vi "NEW LOAD CELL PID.vi"(8 "error in (no error)":errorcluster, 10 "Checkbox":bool, 11 "main ref":T1) -> (0 "error out":errorcluster)   [LabVIEW 2025]
uses:
  controls/LAB-IQ UI Data.ctl
  HEAVE vi's/Heave Write enum.ctl
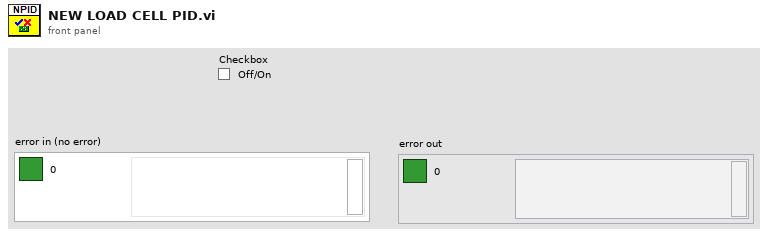
[diagram p1: front panel]
types:
  T1 = typedef "LAB-IQ UI Data.ctl" = cluster{"Main Home Screen":cluster{"GUI":refnum<vi>, "Platform Settings":refnum<vi>, "Configure":refnum<vi>, "Home":refnum<vi>, "EXIT":refnum<vi>, "service 2":refnum<vi>, "MainPage":refnum<vi>, "Analysis":refnum<vi>}, "Platform Settings":cluster{"mm/s  Surge":refnum<vi>, "Update Surge Speed":refnum<vi>, "Drive Error":refnum<vi>, "Disable Axis Jog Soft Limits":refnum<vi>, "mm/s  Sway":refnum<vi>, "Sway and Surge COM Status":refnum<vi>, "Heave COM Status":refnum<vi>, "Enable Platform":refnum<vi>, "Surge Forward Main":refnum<vi>, "Sway Right Main":refnum<vi>, "Sway Left Main":refnum<vi>, "Heave Down Main":refnum<vi>, "Heave Up main":refnum<vi>, "Update Sway Speed":refnum<vi>, "Update Heave Speed":refnum<vi>, "mm/s Heave":refnum<vi>, "mm/sec":refnum<vi>, "mm":refnum<vi>, "Surge Backward Main":refnum<vi>}, "Analysis Screen":cluster{"Analysis Home":refnum<vi>, "Surface Analysis":refnum<vi>, "Imaging":refnum<vi>, "Image Analysis":refnum<vi>, "Post Analysis":refnum<vi>}, "Config Screen":cluster{"Select Load Head":refnum<vi>, "Notes :":refnum<vi>, "FILE":refnum<vi>, "Sample ID :":refnum<vi>, "Operator ID :":refnum<vi>, "Operator Name :":refnum<vi>, "Auto":refnum<vi>}, "Motion Module":cluster{"zNL":refnum<vi>, "NL disp":refnum<vi>, "Rotary Tab":refnum<vi>, "Motion Direction:  3":refnum<vi>, "E.Velocity 2":refnum<vi>, "e.v/ssr 2":refnum<vi>, "Enter Fixed E.Velocity 2":refnum<vi>, "Enter Final SRR 2":refnum<vi>, "Enter initial SRR 2":refnum<vi>, "Enter Fixed SRR 2":refnum<vi>, "Enter the Final E.Velocity (m/s) 2":refnum<vi>, "Enter initial E.Velocity (m/s) 2":refnum<vi>, "Final Speed (RPM) 3":refnum<vi>, "Initial Speed (RPM) 2":refnum<vi>, "Enter the Final Velocity (m/s) 3":refnum<vi>, "Enter initial Velocity (m/s)  3":refnum<vi>, "Ramp Up 2":refnum<vi>, "TEST SELECTION":refnum<vi>, "SPEED SELECTION : ":refnum<vi>, "Angular Oscillation Set":refnum<vi>, "Traction":refnum<vi>, "Step Speed":refnum<vi>, "StepTable For Load-Speed":refnum<vi>, "StepTable For Speed":refnum<vi>, "Surge Forward MM":refnum<vi>, "Surge Backward MM":refnum<vi>, "M3 Image":refnum<vi>, "String 39":refnum<vi>, "Sway Left MM":refnum<vi>, "Sway Right MM":refnum<vi>, "Disable Axis Jog Soft Limits":refnum<vi>, "mm":refnum<vi>, "Heave Down MM":refnum<vi>, "Heave Up MM":refnum<vi>, "Wear Track Diameter (mm)":refnum<vi>, "Set WTD":refnum<vi>, "HomeScratch":refnum<vi>, "HomeRot":refnum<vi>, "PlaceModule":refnum<vi>, "Enter the Angle (Deg)":refnum<vi>, "Enter the Frequency (Hz)":refnum<vi>, "Motion Mode:":refnum<vi>, "LR Sway":refnum<vi>, "Rot Hor":refnum<vi>, "Scratch":refnum<vi>, "LR Cam":refnum<vi>, "MMBack":refnum<vi>, "MMNext":refnum<vi>, "Rot Ver":refnum<vi>, "Rotary Module Selection":refnum<vi>, "calculate rotary":refnum<vi>, "SPEED SELECTION : rotary":refnum<vi>, "Import 2":refnum<vi>, "Save 2":refnum<vi>, "File Path :  2":refnum<vi>, "String 45":refnum<vi>, "StepTable For Speed 3":refnum<vi>, "Enter the Speed(mm/sec)":refnum<vi>, "Enter the Speed(RPM)":refnum<vi>, "Enter Scratch Speed (mm/s):":refnum<vi>, "SwaySpeed Set":refnum<vi>, "Scartch Offset":refnum<vi>, "Motion type:":refnum<vi>, "HomeScratch 2":refnum<vi>, "Enter Scratch length (mm):":refnum<vi>, "Wear Track Diameter":refnum<vi>, "Rotary Speed Exced":refnum<vi>, "Scratch Mode":refnum<vi>, "No of Scratch":refnum<vi>}, "Environmental control":cluster{"Humidity  Status  3":refnum<vi>, "Low Temp  Status  2":refnum<vi>, "TK4 status 2":refnum<vi>, "Stage Temperature":refnum<vi>, "Sample Temperature":refnum<vi>, "Humidity (Amb)":refnum<vi>, "Clear List":refnum<vi>, "Add to list":refnum<vi>, "Wear":refnum<vi>, "Vibration":refnum<vi>, "Humidity (Chamber)":refnum<vi>, "Temperature (Chamber)":refnum<vi>, "ECR ":refnum<vi>, "Temperature (Amb)":refnum<vi>, "Microphone":refnum<vi>, "Acoustic Emission 3":refnum<vi>, "SNext":refnum<vi>, "APBack":refnum<vi>, "Enter the Temperature (°C):":refnum<vi>, "Enter the Stage \nTemperature (°C):":refnum<vi>, "Enter the Humidity (%Rh):":refnum<vi>, "Low Temp":refnum<vi>, "High Temp":refnum<vi>, "Humidity":refnum<vi>, "Sensors Picked":refnum<vi>}, "About Screen":cluster{"Password":refnum<vi>, "Home Service":refnum<vi>, "Advanced Setting":refnum<vi>, "About Tab":refnum<vi>, "ECR Port:":refnum<vi>, "Ramp Port:":refnum<vi>, "Installation/Replacement completed":refnum<vi>, "Loahead":refnum<vi>, "Heave and Surge COM Port:":refnum<vi>, "Sway COM Port:":refnum<vi>, "Temp Modbus:":refnum<vi>, "Humidity Port:":refnum<vi>, "Edit Gain Constants":refnum<vi>, "Save Gain Constants":refnum<vi>}, "Main Screen":cluster{"Main Screen Tab":refnum<vi>, "Angle and Frequency":refnum<vi>, "Stroke (mm)":refnum<vi>, "Angle (Deg)":refnum<vi>, "Main Speed Tab":refnum<vi>, "MTM MOTOR DISPLAY":refnum<vi>, "Disc Speed (m/sec)":refnum<vi>, "Ball Speed (m/sec)":refnum<vi>, "Disc Speed (RPM)":refnum<vi>, "Ball Speed (RPM)":refnum<vi>, "SPEED TAB":refnum<vi>, "Speed (m/sec)":refnum<vi>, "Set Speed (m/sec)":refnum<vi>, "Speed (RPM)":refnum<vi>, "Set Speed":refnum<vi>, "Time Tab":refnum<vi>, "Time ( HH:MM:SS ) 2":refnum<vi>, "Test Duration":refnum<vi>, "Test Duration 4":refnum<vi>, "TEST CYCLE":refnum<vi>, "TOTAL CYCLES":refnum<vi>, "Set Load (N)":refnum<vi>, "Temp Tabs":refnum<vi>, "Heater":refnum<vi>, "TK4 status":refnum<vi>, "ChamberTemp":refnum<vi>, "SetTmp":refnum<vi>, "Controller  Status":refnum<vi>, "ChamberTemp 2":refnum<vi>, "SetTmp 2":refnum<vi>, "Controller  Status 2":refnum<vi>, "ChamberTemp 3":refnum<vi>, "SetTmp 3":refnum<vi>, "Cooling":refnum<vi>, "Load Communication":refnum<vi>, "Ambient \nTemperature":refnum<vi>, "HumCOMStatus":refnum<vi>, "Ambient\n Humidity":refnum<vi>, "Freq (Hz)":refnum<vi>, "Load En":refnum<vi>, "NLt":refnum<vi>, "zNL 2":refnum<vi>, "Humidity On":refnum<vi>, "humidity disp":refnum<vi>, "Set Humidity":refnum<vi>, "NL disp 2":refnum<vi>, "Humidity On 2":refnum<vi>, "humidity disp 2":refnum<vi>, "Set Humidity 2":refnum<vi>, "NL disp 3":refnum<vi>, "AppLoadSeq scratch":refnum<vi>, "Stop Scratch":refnum<vi>, "ClrLog":refnum<vi>, "Trip Log":refnum<vi>, "STOP":refnum<vi>, "Start Test":refnum<vi>, "Test status":refnum<vi>, "AR Led":refnum<vi>, "Data":refnum<vi>, "Health":refnum<vi>, "Sway COM Status":refnum<vi>, "Heave COM Status":refnum<vi>, "Grp Tab":refnum<vi>, "Sub Graph":refnum<vi>, "SD (mm)":refnum<vi>, "Siliding distance Reset Graph":refnum<vi>, "SDGp":refnum<vi>, "Humidity Reset Graph":refnum<vi>, "HumrGp":refnum<vi>, "Acoustic Emission (mV)":refnum<vi>, "Aqucostic Reset Graph":refnum<vi>, "gACQUOS":refnum<vi>, "ECR RESET":refnum<vi>, "ECR":refnum<vi>, "Temperature Reset":refnum<vi>, "Acoustic Emission (mV) 2":refnum<vi>, "Aqucostic Reset Graph 2":refnum<vi>, "gACQUOS 2":refnum<vi>, "ECR RESET 2":refnum<vi>, "ECR 2":refnum<vi>, "Temperature Reset 2":refnum<vi>, "Temperature (deg c)":refnum<vi>, "Speed Reset Graph":refnum<vi>, "Speed Tab":refnum<vi>, "MTM DISC  SPEED":refnum<vi>, "MTM BALL SPEED":refnum<vi>, "speed mm/sec":refnum<vi>, "Hymidity":refnum<vi>, "Humidity Disable trip":refnum<vi>, "CoF Trip  2":refnum<vi>, "Depth Trip":refnum<vi>, "Weart Deapth":refnum<vi>, "Depth Reset Graph":refnum<vi>, "Weart":refnum<vi>, "Depthz":refnum<vi>, "Depth (µm)":refnum<vi>, "WearGp":refnum<vi>, "NL Trip 2":refnum<vi>, "Load pid":refnum<vi>, "Load Disable Trip":refnum<vi>, "Load Reset Graph":refnum<vi>, "NL Display 4":refnum<vi>, "Main Chart 3":refnum<vi>, "BACK":refnum<vi>, "Depth Trip 2":refnum<vi>, "COF TRIP ":refnum<vi>, "Friction Force (N)":refnum<vi>, "FF Reset Graph":refnum<vi>, "FF Disable Trip":refnum<vi>, "FF TRIP":refnum<vi>, "COF Disable Trip":refnum<vi>, "COF Reset Graph":refnum<vi>, "Start Test Temp":refnum<vi>, "zFF":refnum<vi>, "Friction Force (N) Graph":refnum<vi>, "Coefficient of Friction":refnum<vi>, "Scratch Start Test":refnum<vi>, "FF Tab":refnum<vi>, "Cyclic Friction Force (N)":refnum<vi>, "CZ FF":refnum<vi>, "Cyclic Friction Force (N) Graph":refnum<vi>, "Cyclic Coefficient of Friction":refnum<vi>, "Cyclic FF TRIP":refnum<vi>, "Cyclic FF Disable Trip":refnum<vi>, "cyclic COF Disable Trip":refnum<vi>, "cyclic COF TRIP":refnum<vi>, "cyclic COF Reset Graph":refnum<vi>, "Cyclic FF Reset Graph":refnum<vi>, "Test Trip":refnum<vi>, "Multi Scratch Pass":refnum<vi>}, "Loading":cluster{"Indentation":refnum<vi>, "Reference Sample":refnum<vi>, "Load Cell Communication Slide":refnum<vi>, "com 3":refnum<vi>, "com":refnum<vi>, "DecaForce COM Status":refnum<vi>, "Update":refnum<vi>, "Clear 3":refnum<vi>, "seq":refnum<vi>, "Stribeck table":refnum<vi>, "Stribeck Table  For loading":refnum<vi>, "Loading Mode":refnum<vi>, "Enter the Final Load (N)":refnum<vi>, "Enter the CoF Trip":refnum<vi>, "Enter the Friction Force Trip":refnum<vi>, "Enter the Normal load Trip":refnum<vi>, "Enter the Load  (N)":refnum<vi>, "KiloForce":refnum<vi>, "DecaForce ":refnum<vi>, "MicroForce":refnum<vi>, "LHBack":refnum<vi>, "LHNext":refnum<vi>, "Enter the Loading Rate (N/min)":refnum<vi>, "Message":refnum<vi>, "Warning 2":refnum<vi>, "SSP 0.75":refnum<vi>, "SSP 0.5":refnum<vi>, "SSP 0.3":refnum<vi>, "Warning":refnum<vi>, "gui GIF":refnum<vi>, "Communication is established":refnum<vi>, "AppLoad 4":refnum<vi>, "Multipoint":refnum<vi>, "Load Selection":refnum<vi>}, "PID":cluster{"Ramp MulFac":refnum<vi>, "pulses LoadDiffRamp(2..10)":refnum<vi>, "PulseControlRamp(diff<=3N)":refnum<vi>, "SetLoadDeadband(%) Load(0-10N)":refnum<vi>, "PID gains out delay (microForce)":refnum<vi>, "Ramp":refnum<vi>, "Gain 2":refnum<vi>, "pulses LoadDiff(2..10)":refnum<vi>, "pulses LoadDiff(11..50)":refnum<vi>, "PulseControl(diff<=3N)":refnum<vi>, "SetLoadDeadband(%)  2":refnum<vi>, "Dummy Run":refnum<vi>, "Vertical load (N)":refnum<vi>, "AutoTune":refnum<vi>, "Offset 3 ":refnum<vi>, "apply load":refnum<vi>, "Offset  3":refnum<vi>, "apply load 2":refnum<vi>, "Enter ByPass Load":refnum<vi>, "reinit 3":refnum<vi>, "output range delay":refnum<vi>, "PID gains out delay":refnum<vi>, "Bypass Load":refnum<vi>, "pulsesSent":refnum<vi>, "pulses ":refnum<vi>, "actpid":refnum<vi>, "gFF Rot":refnum<vi>, "pulses LoadDiff(21..1000)":refnum<vi>, "Delay":refnum<vi>, "deadband":refnum<vi>}, "Config Parameters":cluster{"Tab Control 3":refnum<vi>, "Tab Control 19":refnum<vi>, "SAMPLES":refnum<vi>, "Re-initilaize":refnum<vi>, "Filter ON/OFF":refnum<vi>, "TracHomeSurgeOffsetCounts 10MM":refnum<vi>, "TracHomeSwayOffsetCounts 10MM":refnum<vi>, "Acoustic Emission:":refnum<vi>, "Apply Filter (FF)":refnum<vi>, "Filter% 2":refnum<vi>, "Apply Filter (Load)":refnum<vi>, "Filter% ":refnum<vi>, "Sway distance (mm)":refnum<vi>, "Surge distance (mm)":refnum<vi>, "DataSavingLoopDelay(ms)":refnum<vi>, "SAVE 2":refnum<vi>, "Enter Distance":refnum<vi>, "Sway Counts:":refnum<vi>, "Distance (mm): 3":refnum<vi>, "Surge Counts:":refnum<vi>, "Distance (mm): 2":refnum<vi>, "Distance (mm):":refnum<vi>, "Heave Counts:":refnum<vi>, "LRMHomeSurgeOffsetCounts":refnum<vi>, "LRMHomeSwayOffsetCounts":refnum<vi>, "TracHomeSurgeOffsetCounts 20MM":refnum<vi>, "TracHomeSwayOffsetCounts 20MM":refnum<vi>, "RotHomeSwayOffsetCounts":refnum<vi>, "RotHomeSurgeOffsetCounts":refnum<vi>, "Heave distance":refnum<vi>, "Zmm":refnum<vi>, "Heave Pulses/mm":refnum<vi>, "Surge Pulses/mm":refnum<vi>, "Sway Pulses/mm":refnum<vi>, "Heave Pitch":refnum<vi>, "Surge Pitch":refnum<vi>, "Sway Pitch":refnum<vi>, "Heave PPR":refnum<vi>, "Surge PPR":refnum<vi>, "Sway PPR":refnum<vi>, "Tab Control 5":refnum<vi>, "Tab Control 14":refnum<vi>, "Tab Control 26":refnum<vi>, "AE":refnum<vi>, "Heave Loop Delay":refnum<vi>, "Heave PID Speed":refnum<vi>, "Surge Jog Speed":refnum<vi>, "Heave Jog Speed":refnum<vi>, "Sway Loop Delay":refnum<vi>, "Sway PID Speed":refnum<vi>, "Sway Jog Speed":refnum<vi>}, "Loading Com Port":cluster{"ClearAll":refnum<vi>, "Mz(Nm)":refnum<vi>, "My(Nm)":refnum<vi>, "Mx(Nm)":refnum<vi>, "Save Dwell":refnum<vi>, "Mx ":refnum<vi>, "My ":refnum<vi>, "Mz":refnum<vi>, "Fx(N)":refnum<vi>, "Fy(N)":refnum<vi>, "Fz(N)":refnum<vi>, "ZeroAll":refnum<vi>, "Acq Delay (ms)":refnum<vi>, "Burst Delay (ms)":refnum<vi>, "model":refnum<vi>, "SN":refnum<vi>, "FFx(N)":refnum<vi>, "Sensor IP":refnum<vi>, "Port":refnum<vi>, "FFy(N)":refnum<vi>, "Load(N)":refnum<vi>, "delete Handle":refnum<vi>, "Create Handle":refnum<vi>, "ft_data":refnum<vi>, "ft_range":refnum<vi>, "ft_data 2":refnum<vi>, "stop 6":refnum<vi>, "running_flag":refnum<vi>, "ft_udp_handle":refnum<vi>, "get-data-return":refnum<vi>, "get-range-return":refnum<vi>, "zero-return":refnum<vi>, "filter-return":refnum<vi>, "initial-return":refnum<vi>, "deleteHandle-result":refnum<vi>, "Load Cell Temp":refnum<vi>}, "Heave AND Surge":cluster{"SURGE POSE":refnum<vi>, "error out Read":refnum<vi>, "HEAVE POSE":refnum<vi>, "State":refnum<vi>, "Homed":refnum<vi>, "Sequence ID":refnum<vi>, "error out Write":refnum<vi>, "faultCode":refnum<vi>, "Ack ID":refnum<vi>, "SPEED":refnum<vi>, "Distance":refnum<vi>, "Mode Command":refnum<vi>, "Heave and Surge Read":refnum<vi>, "Read Heave Temp":refnum<vi>, "Spare 15":refnum<vi>, "Spare 14":refnum<vi>, "Spare 13":refnum<vi>, "Spare 12":refnum<vi>, "Spare 11":refnum<vi>, "Spare 10":refnum<vi>, "Spare 9":refnum<vi>, "Spare 8":refnum<vi>, "Spare 7":refnum<vi>, "Spare 6":refnum<vi>, "Spare 5":refnum<vi>, "Spare 4":refnum<vi>, "Spare 2":refnum<vi>, "Spare 1":refnum<vi>, "Node Id":refnum<vi>, "Spare 3":refnum<vi>, "SPARE 4":refnum<vi>, "SPARE 3":refnum<vi>, "SPARE 2":refnum<vi>, "SPARE 1":refnum<vi>, "fwMajor":refnum<vi>, "fwMinor":refnum<vi>, "Manual Write":refnum<vi>, "Heave and Surge Write":refnum<vi>}, "New PID LOGIC":cluster{"Fine Tune Zone":refnum<vi>, "PID SDelay":refnum<vi>, "Max_pos_limit":refnum<vi>, "Min_pos_limit":refnum<vi>, "i_limit":refnum<vi>, "pct_scale":refnum<vi>, "Deadband":refnum<vi>, "Kd":refnum<vi>, "Ki":refnum<vi>, "Kp":refnum<vi>, "Current Position":refnum<vi>, "Set Load":refnum<vi>, "Current Load":refnum<vi>, "Pulse delta":refnum<vi>, "Init Step":refnum<vi>, "Max Step Linit":refnum<vi>}, "SWAY ":cluster{"fwMajor":refnum<vi>, "Homed":refnum<vi>, "Rotary POSE":refnum<vi>, "State":refnum<vi>, "SWAY POSE":refnum<vi>, "Ack ID":refnum<vi>, "faultCode":refnum<vi>, "Node Id":refnum<vi>, "fwMinor":refnum<vi>, "Spare 6":refnum<vi>, "Spare 5":refnum<vi>, "Spare 4":refnum<vi>, "Spare 3":refnum<vi>, "Spare 2":refnum<vi>, "Spare 1":refnum<vi>, "Spare 7":refnum<vi>, "SPARE  5":refnum<vi>, "error out Write  SWAY ":refnum<vi>, "error out Read SWAY ":refnum<vi>, "Manual Write SWAY ":refnum<vi>, "SWAY WRITE":refnum<vi>, "SPARE  4":refnum<vi>, "SPARE  3":refnum<vi>, "SPARE 2":refnum<vi>, "SPARE 1":refnum<vi>, "Spare 15":refnum<vi>, "Spare 14":refnum<vi>, "Spare 13":refnum<vi>, "Spare 12":refnum<vi>, "Spare 11":refnum<vi>, "Spare 9":refnum<vi>, "Spare 8":refnum<vi>, "SPEED":refnum<vi>, "Distance":refnum<vi>, "Mode Command":refnum<vi>, "Sequence ID":refnum<vi>, "SWAY READ":refnum<vi>, "Spare 10":refnum<vi>, "Read SWAY Temp":refnum<vi>}, "Analysis Screen":cluster{"Analysis Home":refnum<vi>, "Refresh 2":refnum<vi>, "MEAN 4":refnum<vi>, "SD 4":refnum<vi>, "VARIANCE 4":refnum<vi>, "MEAN  3":refnum<vi>, "SD  3":refnum<vi>, "VARIANCE  3":refnum<vi>, "MEAN 2":refnum<vi>, "SD  2":refnum<vi>, "VARIANCE 2":refnum<vi>, "MEAN":refnum<vi>, "SD":refnum<vi>, "VARIANCE":refnum<vi>, "File 4 Discription":refnum<vi>, "OPEN 4":refnum<vi>, "File Name 4":refnum<vi>, "OPEN 3":refnum<vi>, "File 3 Discription":refnum<vi>, "File Name 3":refnum<vi>, "Y-AXIS":refnum<vi>, "X-AXIS":refnum<vi>, "XY Graph":refnum<vi>, "File Name 2":refnum<vi>, "File Name 1":refnum<vi>, "OPEN 2":refnum<vi>, "OPEN 1":refnum<vi>, "File 1 Discription ":refnum<vi>, "File 2 Discription":refnum<vi>}}
  T2 = typedef "Heave Write enum.ctl" = enum16{"INIT", "WRITE", "CLOSE", "REINIT"}
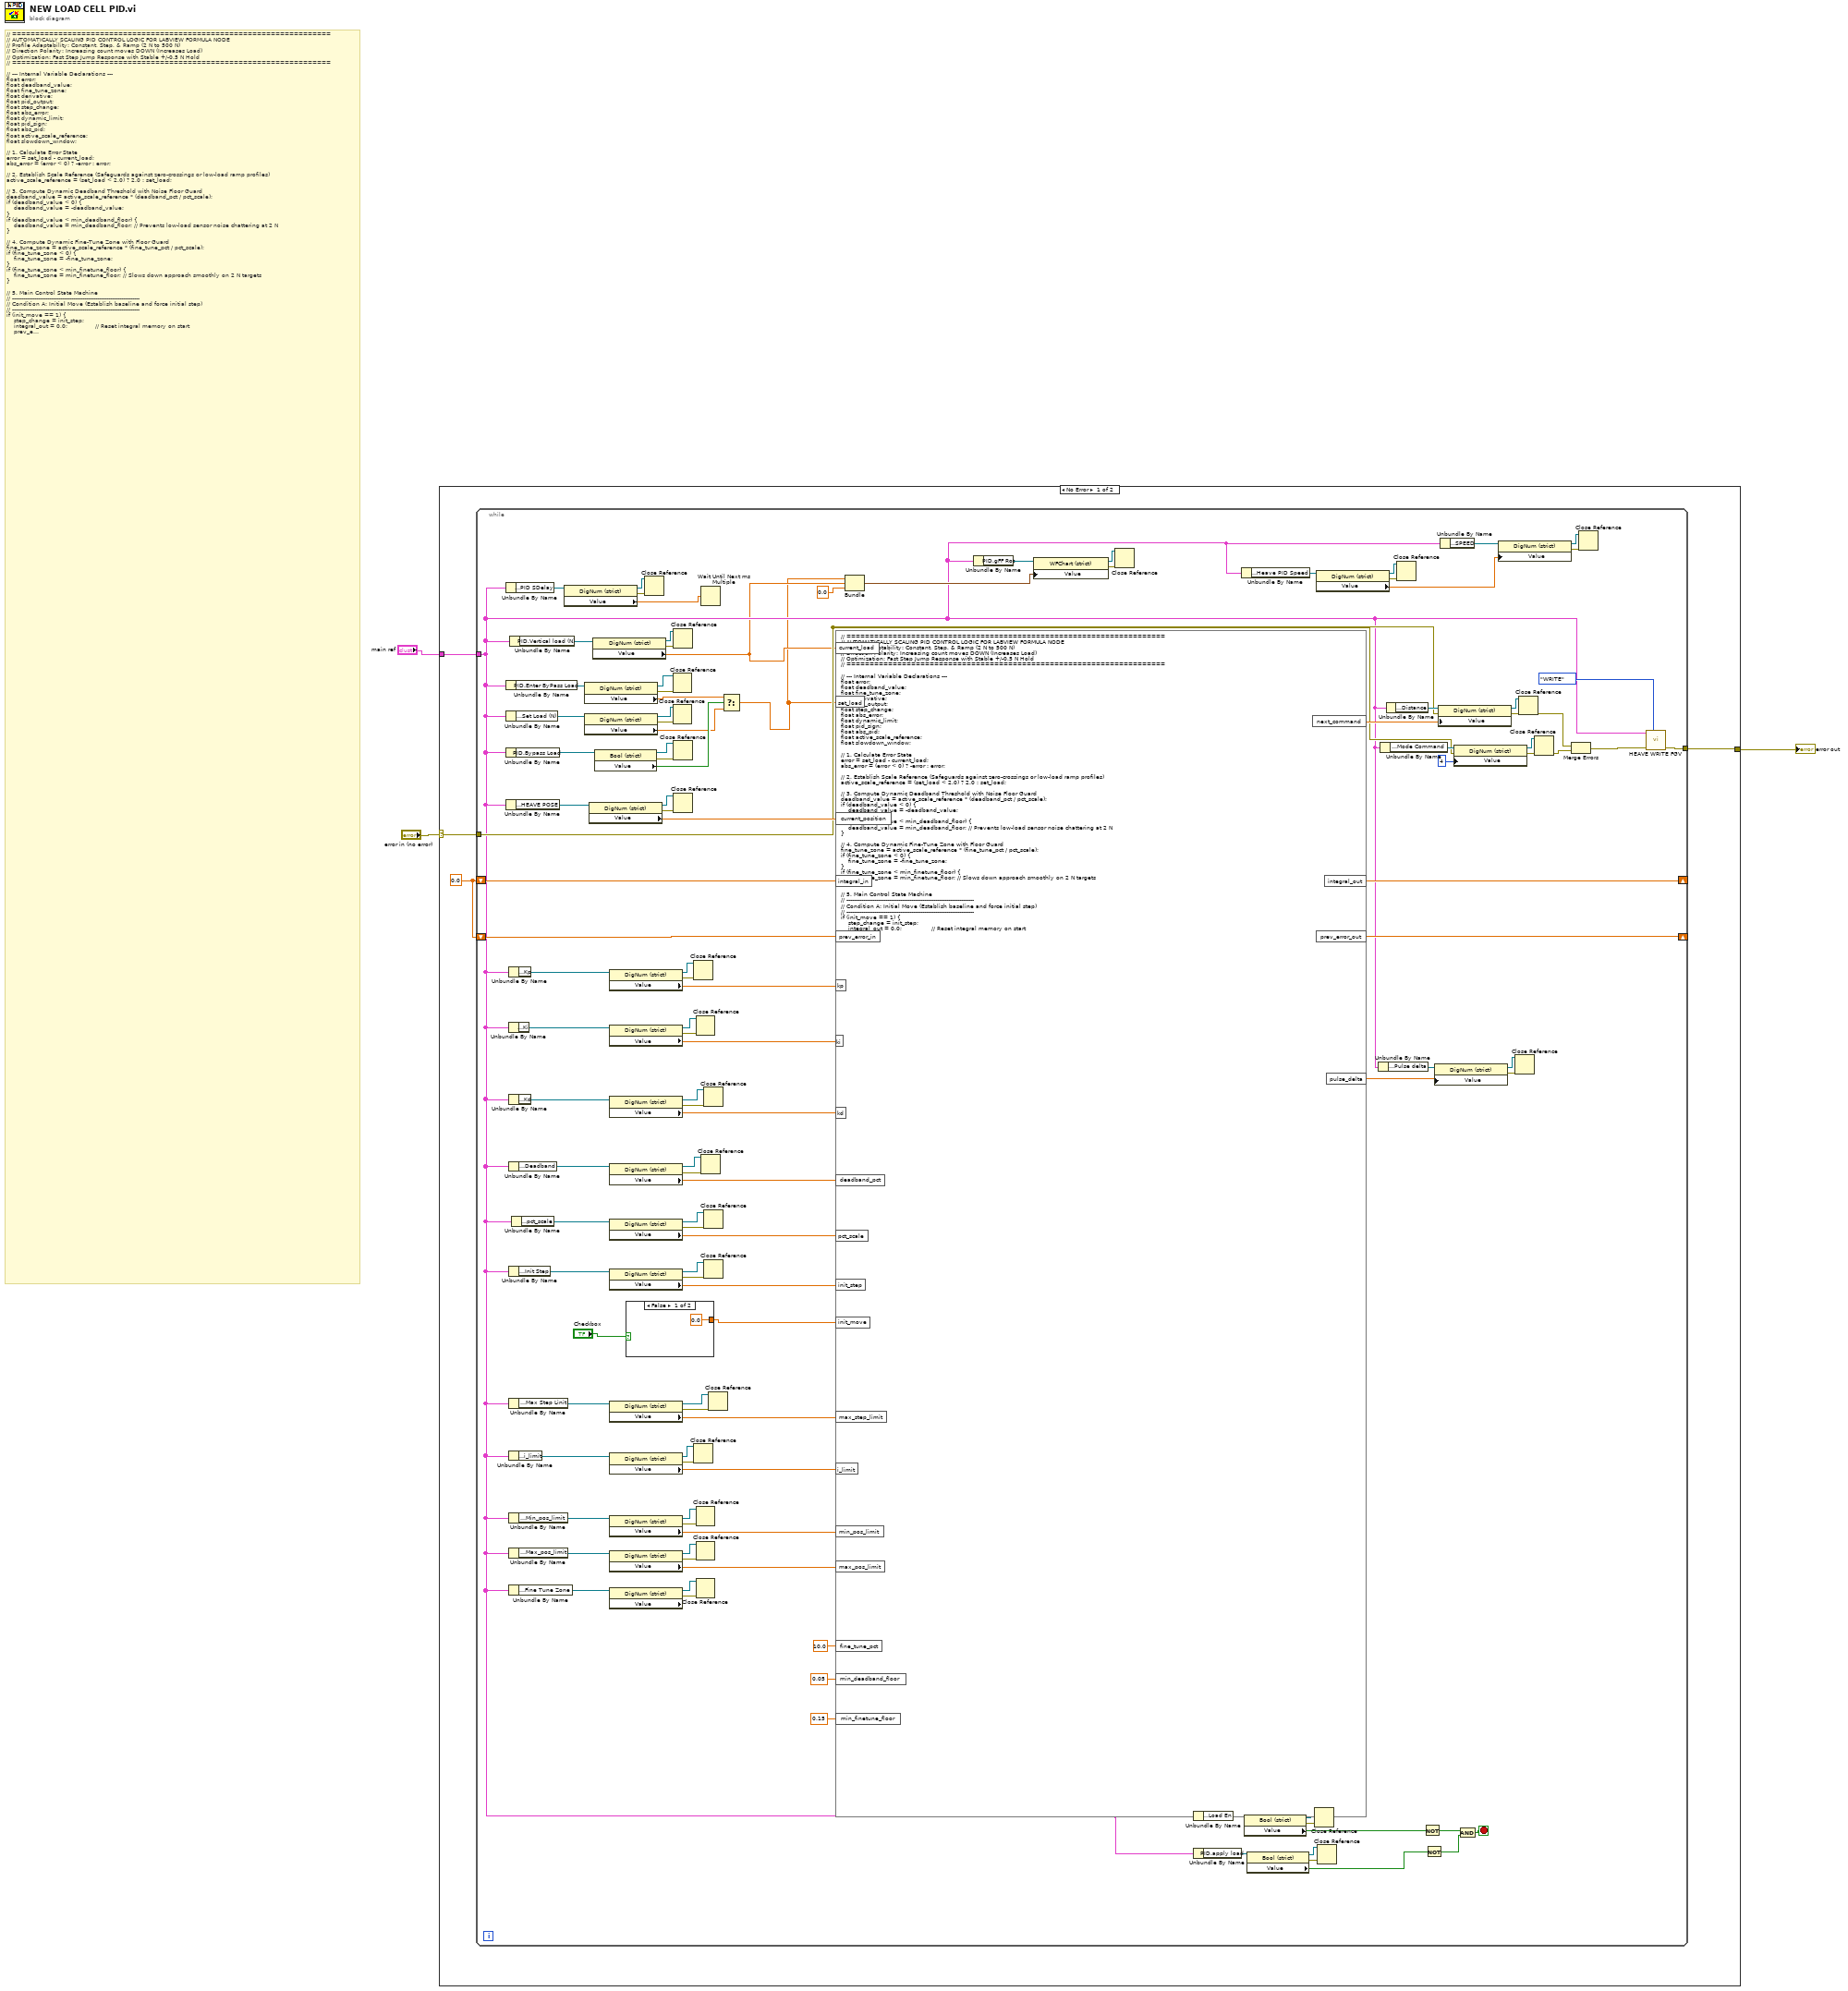
[diagram p0: block diagram]
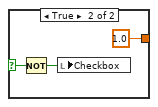
[diagram p2: hidden frame]
diagram:
  # "// =====================================================================\n// AUTOMATICALLY SCALING PID CONTROL LOGIC FOR LABVIEW FORMULA NODE\n// Profile Adaptability: Constant, Step, & Ramp (2 N to 500 N)\n// Direction Polarity: Increasing count moves DOWN (Increases Load)\n// Optimization: Fast Step Jump Response with Stable +/-0.5 N Hold\n// =====================================================================\n\n// --- Internal Variable Declarations ---\nfloat error;\nfloat deadband_value;\nfloat fine_tune_zone;\nfloat derivative;\nfloat pid_output;\nfloat step_change;\nfloat abs_error;\nfloat dynamic_limit;\nfloat pid_sign;\nfloat abs_pid;\nfloat active_scale_reference;\nfloat slowdown_window;\n\n// 1. Calculate Error State\nerror = set_load - current_load;\nabs_error = (error < 0) ? -error : error;\n\n// 2. Establish Scale Reference (Safeguards against zero-crossings or low-load ramp profiles)\nactive_scale_reference = (set_load < 2.0) ? 2.0 : set_load;\n\n// 3. Compute Dynamic Deadband Threshold with Noise Floor Guard\ndeadband_value = active_scale_reference * (deadband_pct / pct_scale);\nif (deadband_value < 0) {\n    deadband_value = -deadband_value; \n}\nif (deadband_value < min_deadband_floor) {\n    deadband_value = min_deadband_floor; // Prevents low-load sensor noise chattering at 2 N\n}\n\n// 4. Compute Dynamic Fine-Tune Zone with Floor Guard\nfine_tune_zone = active_scale_reference * (fine_tune_pct / pct_scale);\nif (fine_tune_zone < 0) {\n    fine_tune_zone = -fine_tune_zone;\n}\nif (fine_tune_zone < min_finetune_floor) {\n    fine_tune_zone = min_finetune_floor; // Slows down approach smoothly on 2 N targets\n}\n\n// 5. Main Control State Machine\n// ---------------------------------------------------------------------\n// Condition A: Initial Move (Establish baseline and force initial step)\n// ---------------------------------------------------------------------\nif (init_move == 1) {\n    step_change = init_step; \n    integral_out = 0.0;               // Reset integral memory on start\n    prev_error_out = error;           // Initialize derivative baseline\n    \n    if (error > 0) {\n        next_command = current_position + step_change;\n    } else {\n        next_command = current_position - step_change;\n    }\n    pulse_delta = next_command - current_position;\n}\n// ---------------------------------------------------------------------\n// Condition B: Within Target Deadband (Freeze State / Zero Energy Output)\n// ---------------------------------------------------------------------\nelse if (abs_error <= deadband_value) {\n    step_change = 0.0;\n    next_command = current_position;  // Lock to current physical position\n    integral_out = integral_in;       // Freeze integral to prevent drift\n    prev_error_out = error;           // Keep derivative baseline fresh\n    pulse_delta = 0.0;                // Zero pulse execution to kill motor energy completely\n} \n// ---------------------------------------------------------------------\n// Condition C: Active PID Control Zone\n// ---------------------------------------------------------------------\nelse {\n    // A. Track Integral with strict Anti-Windup Limits\n    integral_out = integral_in + error;\n    if (integral_out > i_limit) {\n        integral_out = i_limit;\n    } else if (integral_out < -i_limit) {\n        integral_out = -i_limit;\n    }\n\n    // B. Calculate Derivative (Tracks rate of change of error - crucial for RAMP tracking)\n    derivative = error - prev_error_in;\n    prev_error_out = error; \n\n    // C. Execute Raw PID Equation\n    pid_output = (error * kp) + (integral_out * ki) + (derivative * kd);\n    \n    // D. Extract Mathematical Sign and Magnitude\n    pid_sign = (pid_output >= 0) ? 1.0 : -1.0;\n    abs_pid = (pid_output < 0) ? -pid_output : pid_output;\n\n    // E. Continuous Linear Ramp-Down Ceiling (Optimized for Fast Step & Tight Hold)\n    // Limits slowdown behavior exclusively to a 2.0 N window near the target load\n    slowdown_window = 2.0; \n\n    if (abs_error < slowdown_window) {\n        dynamic_limit = max_step_limit * (abs_error / slowdown_window);\n        if (dynamic_limit < 1.0) {\n            dynamic_limit = 1.0; // Minimum microstep velocity floor\n        }\n    } else {\n        dynamic_limit = max_step_limit; // Full throttle speed allowed for high error step jumps\n    }\n\n    // F. Apply Smooth Step Control & Fine Tuning Zone\n    // Aligned perfectly to your +/-0.5 N hold requirement\n    if (abs_error <= 0.5) {\n        step_change = 1.0; // Minimal 1-count micro-stepping to lock firmly onto target\n    } else {\n        if (abs_pid < dynamic_limit) {\n            step_change = abs_pid; // Decay step size perfectly near steady state\n        } else {\n            step_change = dynamic_limit; // Cap velocity ceiling to prevent overshooting\n        }\n    }\n    \n    // G. Apply Step Vector directly relative to physical position\n    next_command = current_position + (step_change * pid_sign);\n    pulse_delta = next_command - current_position;\n}\n\n// 6. Hard Structural Boundaries & Safety Guards\n// ---------------------------------------------------------------------\nif (next_command > max_pos_limit) {\n    next_command = max_pos_limit;\n    pulse_delta = next_command - current_position;\n} else if (next_command < min_pos_limit) {\n    next_command = min_pos_limit;\n    pulse_delta = next_command - current_position;\n}"
  n1 = case shown="No Error" "error in (no error)" {
    selector: "error in (no error)" -> [w5 _]
    tunnel: "main ref" -> [w7 _]
    tunnel: [w4 _] -> w1
    frame No Error {
      w6 = 0.0
      n2 = while {
        tunnel: w7 -> [w15]
        shift-right: [w49] -> _
        shift-left: w6 -> [w96]
        shift-right: [w48] -> _
        shift-left: w6 -> [w95]
        tunnel: w5 -> [w28]
        tunnel: [w24] -> w4
        stop <- w113 stop-if-true
        n3 = Unbundle By Name(w15) -> ("New PID LOGIC.PID SDelay"=w124:refnum<vi>)
        n4 = Unbundle By Name(w15) -> ("PID.Enter ByPass Load"=w109:refnum<vi>)
        n5 = Unbundle By Name(w15) -> ("Main Screen.Set Load (N)"=w117:refnum<vi>)
        n6 = Unbundle By Name(w15) -> ("PID.Bypass Load"=w104:refnum<vi>)
        n7 = Unbundle By Name(w15) -> ("Heave AND Surge.HEAVE POSE"=w100:refnum<vi>)
        n8 = Unbundle By Name(w15) -> ("New PID LOGIC.Kp"=w94:refnum<vi>)
        n9 = Unbundle By Name(w15) -> ("New PID LOGIC.Ki"=w88:refnum<vi>)
        n10 = Unbundle By Name(w15) -> ("New PID LOGIC.Kd"=w86:refnum<vi>)
        n11 = Unbundle By Name(w15) -> ("New PID LOGIC.Deadband"=w80:refnum<vi>)
        n12 = Unbundle By Name(w15) -> ("New PID LOGIC.Init Step"=w72:refnum<vi>)
        n13 = Unbundle By Name(w15) -> ("New PID LOGIC.Max Step Linit"=w68:refnum<vi>)
        n14 = Unbundle By Name(w15) -> ("New PID LOGIC.i_limit"=w62:refnum<vi>)
        n15 = Unbundle By Name(w15) -> ("New PID LOGIC.Min_pos_limit"=w60:refnum<vi>)
        n16 = Unbundle By Name(w15) -> ("New PID LOGIC.Max_pos_limit"=w54:refnum<vi>)
        n17 = Unbundle By Name(w15) -> ("New PID LOGIC.Fine Tune Zone"=w52:refnum<vi>)
        n18 = Unbundle By Name(w15) -> ("PID.Vertical load (N)"=w14:refnum<vi>)
        n19 = Unbundle By Name(w15) -> ("New PID LOGIC.pct_scale"=w78:refnum<vi>)
        n20 = property class="DigNum (strict)"(reference=w124) -> (reference out=w126:refnum<vi>, error out=w125:errorcluster, "Value"=w123:dbl)  [unwired: 1 in]
        n21 = property class="DigNum (strict)"(reference=w109) -> (reference out=w107:refnum<vi>, error out=w108:errorcluster, "Value"=w102:dbl)  [unwired: 1 in]
        n22 = property class="DigNum (strict)"(reference=w117) -> (reference out=w119:refnum<vi>, error out=w118:errorcluster, "Value"=w101:dbl)  [unwired: 1 in]
        n23 = property class="DigNum (strict)"(reference=w100) -> (reference out=w98:refnum<vi>, error out=w99:errorcluster, "Value"=w97:sgl)  [unwired: 1 in]
        n24 = property class="DigNum (strict)"(reference=w14) -> (reference out=w16:refnum<vi>, error out=w17:errorcluster, "Value"=w9:dbl)  [unwired: 1 in]
        n25 = property class="Bool (strict)"(reference=w104) -> (reference out=w106:refnum<vi>, error out=w105:errorcluster, "Value"=w103:bool)  [unwired: 1 in]
        n26 = property class="DigNum (strict)"(reference=w94) -> (reference out=w92:refnum<vi>, error out=w93:errorcluster, "Value"=w91:dbl)  [unwired: 1 in]
        n27 = property class="DigNum (strict)"(reference=w88) -> (reference out=w90:refnum<vi>, error out=w89:errorcluster, "Value"=w87:dbl)  [unwired: 1 in]
        n28 = property class="DigNum (strict)"(reference=w86) -> (reference out=w84:refnum<vi>, error out=w85:errorcluster, "Value"=w83:dbl)  [unwired: 1 in]
        n29 = property class="DigNum (strict)"(reference=w80) -> (reference out=w82:refnum<vi>, error out=w81:errorcluster, "Value"=w79:dbl)  [unwired: 1 in]
        n30 = property class="DigNum (strict)"(reference=w78) -> (reference out=w76:refnum<vi>, error out=w77:errorcluster, "Value"=w75:dbl)  [unwired: 1 in]
        n31 = property class="DigNum (strict)"(reference=w72) -> (reference out=w74:refnum<vi>, error out=w73:errorcluster, "Value"=w71:dbl)  [unwired: 1 in]
        n32 = property class="DigNum (strict)"(reference=w68) -> (reference out=w66:refnum<vi>, error out=w67:errorcluster, "Value"=w65:dbl)  [unwired: 1 in]
        n33 = property class="DigNum (strict)"(reference=w62) -> (reference out=w64:refnum<vi>, error out=w63:errorcluster, "Value"=w61:dbl)  [unwired: 1 in]
        n34 = property class="DigNum (strict)"(reference=w60) -> (reference out=w58:refnum<vi>, error out=w59:errorcluster, "Value"=w57:dbl)  [unwired: 1 in]
        n35 = property class="DigNum (strict)"(reference=w54) -> (reference out=w56:refnum<vi>, error out=w55:errorcluster, "Value"=w53:dbl)  [unwired: 1 in]
        n36 = property class="DigNum (strict)" props=["Value"](reference=w52) -> (reference out=w50:refnum<vi>, error out=w51:errorcluster)  [unwired: 1 in, 1 out]
        n37 = case shown="False" "Checkbox" {
          selector: "Checkbox" -> [_ w130]
          tunnel: [0.0 1.0] -> w69
          frame False {
          }
          frame True {
            n38 = Not(x=w130) -> (.not. x?=w129:bool)
            n39 = local write "Checkbox"(w129) -> ()
          }
        }
        n40 = Close Reference(reference=w126, error in (no error)=w125) -> ()  [unwired: 1 out]
        n41 = Close Reference(reference=w107, error in (no error)=w108) -> ()  [unwired: 1 out]
        n42 = Close Reference(reference=w119, error in (no error)=w118) -> ()  [unwired: 1 out]
        n43 = Close Reference(reference=w16, error in (no error)=w17) -> ()  [unwired: 1 out]
        n44 = Close Reference(reference=w106, error in (no error)=w105) -> ()  [unwired: 1 out]
        n45 = Close Reference(reference=w98, error in (no error)=w99) -> ()  [unwired: 1 out]
        n46 = Close Reference(reference=w92, error in (no error)=w93) -> ()  [unwired: 1 out]
        n47 = Close Reference(reference=w64, error in (no error)=w63) -> ()  [unwired: 1 out]
        n48 = Close Reference(reference=w90, error in (no error)=w89) -> ()  [unwired: 1 out]
        n49 = Close Reference(reference=w58, error in (no error)=w59) -> ()  [unwired: 1 out]
        n50 = Close Reference(reference=w56, error in (no error)=w55) -> ()  [unwired: 1 out]
        n51 = Close Reference(reference=w50, error in (no error)=w51) -> ()  [unwired: 1 out]
        n52 = Wait Until Next ms Multiple(millisecond multiple=w123) -> ()  [unwired: 1 out]
        n53 = Close Reference(reference=w82, error in (no error)=w81) -> ()  [unwired: 1 out]
        n54 = Close Reference(reference=w84, error in (no error)=w85) -> ()  [unwired: 1 out]
        n55 = Close Reference(reference=w76, error in (no error)=w77) -> ()  [unwired: 1 out]
        n56 = Close Reference(reference=w74, error in (no error)=w73) -> ()  [unwired: 1 out]
        n57 = Close Reference(reference=w66, error in (no error)=w67) -> ()  [unwired: 1 out]
        n58 = Select(t=w102, s=w103, f=w101) -> (s? t:f=w8:dbl)
        n59 = formula code="// =====================================================================\n// AUTOMATICALLY SCALING PID CONTROL LOGIC FOR LABVIEW FORMULA NODE\n// Profile Adaptability: Constant, Step, & Ramp (2 N to 500 N)\n// Direction Polarity: Increasing count moves DOWN (Increases Load)\n// Optimization: Fast Step Jump Response with Stable +/-0.5 N Hold\n// =====================================================================\n\n// --- Internal Variable Declarations ---\nfloat error;\nfloat deadband_value;\nfloat fine_tune_zone;\nfloat derivative;\nfloat pid_output;\nfloat step_change;\nfloat abs_error;\nfloat dynamic_limit;\nfloat pid_sign;\nfloat abs_pid;\nfloat active_scale_reference;\nfloat slowdown_window;\n\n// 1. Calculate Error State\nerror = set_load - current_load;\nabs_error = (error < 0) ? -error : error;\n\n// 2. Establish Scale Reference (Safeguards against zero-crossings or low-load ramp profiles)\nactive_scale_reference = (set_load < 2.0) ? 2.0 : set_load;\n\n// 3. Compute Dynamic Deadband Threshold with Noise Floor Guard\ndeadband_value = active_scale_reference * (deadband_pct / pct_scale);\nif (deadband_value < 0) {\n    deadband_value = -deadband_value; \n}\nif (deadband_value < min_deadband_floor) {\n    deadband_value = min_deadband_floor; // Prevents low-load sensor noise chattering at 2 N\n}\n\n// 4. Compute Dynamic Fine-Tune Zone with Floor Guard\nfine_tune_zone = active_scale_reference * (fine_tune_pct / pct_scale);\nif (fine_tune_zone < 0) {\n    fine_tune_zone = -fine_tune_zone;\n}\nif (fine_tune_zone < min_finetune_floor) {\n    fine_tune_zone = min_finetune_floor; // Slows down approach smoothly on 2 N targets\n}\n\n// 5. Main Control State Machine\n// ---------------------------------------------------------------------\n// Condition A: Initial Move (Establish baseline and force initial step)\n// ---------------------------------------------------------------------\nif (init_move == 1) {\n    step_change = init_step; \n    integral_out = 0.0;                // Reset integral memory on start\n    prev_error_out = error;            // Initialize derivative baseline\n    \n    if (error > 0) {\n        next_command = current_position + step_change;\n    } else {\n        next_command = current_position - step_change;\n    }\n    pulse_delta = next_command - current_position;\n}\n// ---------------------------------------------------------------------\n// Condition B: Within Target Deadband (Freeze State / Zero Energy Output)\n// ---------------------------------------------------------------------\nelse if (abs_error <= deadband_value) {\n    step_change = 0.0;\n    next_command = current_position;  // Lock to current physical position\n    integral_out = integral_in;       // Freeze integral to prevent drift\n    prev_error_out = error;           // Keep derivative baseline fresh\n    pulse_delta = 0.0;                 // Zero pulse execution to kill motor energy completely\n} \n// ---------------------------------------------------------------------\n// Condition C: Active PID Control Zone\n// ---------------------------------------------------------------------\nelse {\n    // A. Track Integral with strict Anti-Windup Limits\n    integral_out = integral_in + error;\n    if (integral_out > i_limit) {\n        integral_out = i_limit;\n    } else if (integral_out < -i_limit) {\n        integral_out = -i_limit;\n    }\n\n    // B. Calculate Derivative (Tracks rate of change of error - crucial for RAMP tracking)\n    derivative = error - prev_error_in;\n    prev_error_out = error; \n\n    // C. Execute Raw PID Equation\n    pid_output = (error * kp) + (integral_out * ki) + (derivative * kd);\n    \n    // D. Extract Mathematical Sign and Magnitude\n    pid_sign = (pid_output >= 0) ? 1.0 : -1.0;\n    abs_pid = (pid_output < 0) ? -pid_output : pid_output;\n\n    // E. Continuous Linear Ramp-Down Ceiling (Optimized for Fast Step & Tight Hold)\n    // Limits slowdown behavior exclusively to a 2.0 N window near the target load\n    slowdown_window = 2.0; \n\n    if (abs_error < slowdown_window) {\n        dynamic_limit = max_step_limit * (abs_error / slowdown_window);\n        if (dynamic_limit < 1.0) {\n            dynamic_limit = 1.0; // Minimum microstep velocity floor\n        }\n    } else {\n        dynamic_limit = max_step_limit; // Full throttle speed allowed for high error step jumps\n    }\n\n    // F. Apply Smooth Step Control & Fine Tuning Zone\n    // Aligned perfectly to your +/-0.5 N hold requirement\n    if (abs_error <= 0.5) {\n        step_change = 1.0; // Minimal 1-count micro-stepping to lock firmly onto target\n    } else {\n        if (abs_pid < dynamic_limit) {\n            step_change = abs_pid; // Decay step size perfectly near steady state\n        } else {\n            step_change = dynamic_limit; // Cap velocity ceiling to prevent overshooting\n        }\n    }\n    \n    // --- CRITICAL ADDITION: Minimum Physical Pulse Guard ---\n    // If active control demands a move, force it to meet your hardware's 1-pulse minimum limit\n    if (step_change < 1.0) {\n        step_change = 1.0;\n    }\n    \n    // G. Apply Step Vector directly relative to physical position\n    next_command = current_position + (step_change * pid_sign);\n    pulse_delta = next_command - current_position;\n}\n\n// 6. Hard Structural Boundaries & Safety Guards\n// ---------------------------------------------------------------------\nif (next_command > max_pos_limit) {\n    next_command = max_pos_limit;\n    pulse_delta = next_command - current_position;\n} else if (next_command < min_pos_limit) {\n    next_command = min_pos_limit;\n    pulse_delta = next_command - current_position;\n}"("current_load"=w9, "set_load"=w8, "current_position"=w97, "integral_in"=w96, "prev_error_in"=w95, "kp"=w91, "ki"=w87, "kd"=w83, "deadband_pct"=w79, "pct_scale"=w75, "init_step"=w71, "init_move"=w69, "max_step_limit"=w65, "i_limit"=w61, "min_pos_limit"=w57, "max_pos_limit"=w53, "fine_tune_pct"=10.0 ("input variable"), "min_deadband_floor"=0.05 ("input variable"), "min_finetune_floor"=0.15 ("input variable")) -> ("next_command"=w40:dbl, "integral_out"=w49:dbl, "prev_error_out"=w48:dbl, "pulse_delta"=w44:dbl)
        n60 = Bundle("Value"=w8, "Value"=w9, 0.0) -> (w19:cluster{"Value":dbl, "Value":dbl, dbl})  [unwired: 1 in]
        n61 = Unbundle By Name(w15) -> ("PID.gFF Rot"=w20:refnum<vi>)
        n62 = property class="WFChart (strict)"(reference=w20, "Value"=w19) -> (reference out=w22:refnum<vi>, error out=w21:errorcluster)  [unwired: 1 in]
        n63 = Close Reference(reference=w22, error in (no error)=w21) -> ()  [unwired: 1 out]
        n64 = Unbundle By Name(w15) -> ("Main Screen.Load En"=w122:refnum<vi>)
        n65 = Unbundle By Name(w15) -> ("PID.apply load"=w114:refnum<vi>)
        n66 = Unbundle By Name(w15) -> ("Config Parameters.Heave PID Speed"=w30:refnum<vi>)
        n67 = property class="Bool (strict)"(reference=w122) -> (reference out=w120:refnum<vi>, error out=w121:errorcluster, "Value"=w10:bool)  [unwired: 1 in]
        n68 = property class="Bool (strict)"(reference=w114) -> (reference out=w116:refnum<vi>, error out=w115:errorcluster, "Value"=w111:bool)  [unwired: 1 in]
        n69 = Close Reference(reference=w120, error in (no error)=w121) -> ()  [unwired: 1 out]
        n70 = property class="DigNum (strict)"(reference=w30) -> (reference out=w32:refnum<vi>, error out=w31:errorcluster, "Value"=w29:dbl)  [unwired: 1 in]
        n71 = Close Reference(reference=w116, error in (no error)=w115) -> ()  [unwired: 1 out]
        n72 = Unbundle By Name(w15) -> ("New PID LOGIC.Pulse delta"=w47:refnum<vi>)
        n73 = Unbundle By Name(w15) -> ("Heave AND Surge.Mode Command"=w37:refnum<vi>)
        n74 = Unbundle By Name(w15) -> ("Heave AND Surge.Distance"=w43:refnum<vi>)
        n75 = Close Reference(reference=w32, error in (no error)=w31) -> ()  [unwired: 1 out]
        n76 = Not(x=w10) -> (.not. x?=w112:bool)
        n77 = Not(x=w111) -> (.not. x?=w110:bool)
        n78 = property class="DigNum (strict)"(reference=w47, "Value"=w44) -> (reference out=w45:refnum<vi>, error out=w46:errorcluster)  [unwired: 1 in]
        n79 = property class="DigNum (strict)"(reference=w43, error in=w28, "Value"=w40) -> (reference out=w41:refnum<vi>, error out=w42:errorcluster)
        n80 = Unbundle By Name(w15) -> ("Heave AND Surge.SPEED"=w35:refnum<vi>)
        n81 = property class="DigNum (strict)"(reference=w37, error in=w28, "Value"=u8 4) -> (reference out=w39:refnum<vi>, error out=w38:errorcluster)
        n82 = And(x=w112, y=w110) -> (x .and. y?=w113:bool)
        n83 = property class="DigNum (strict)"(reference=w35, "Value"=w29) -> (reference out=w33:refnum<vi>, error out=w34:errorcluster)  [unwired: 1 in]
        n84 = Close Reference(reference=w45, error in (no error)=w46) -> ()  [unwired: 1 out]
        n85 = Close Reference(reference=w41, error in (no error)=w42) -> (error out=w25:errorcluster)
        n86 = Close Reference(reference=w39, error in (no error)=w38) -> (error out=w27:errorcluster)
        n87 = Merge Errors(w25, w27) -> (w26:errorcluster)
        n88 = Close Reference(reference=w33, error in (no error)=w34) -> ()  [unwired: 1 out]
        n89 = call "HEAVE WRITE FGV.vi"("Enum - Menu"=Heave_Write_enum."WRITE", "error in (no error)"=w26, "main ref"=w15) -> ("error out"=w24:errorcluster)  [unwired: 8 in]
      }
    }
    frame Error {
    }
  }
  "error out" <- w1
